vi "E709_Sample_Application_1.vi"() -> ()   [LabVIEW 2014, in "PiFOC.lvlib"]
doc: "This VI demonstrates how to initialize an E-709 system, how to move the axis and how to query for the position value of the axis. \n\nIn this example the E-709 is connected through COM port 1 with baudrate 115200. The VI runs E709_Configuration_Setup.vi with these specified settings, moves the axis relative to its current position and reads the position of the axis. The diagram shows how to combine the driver VIs for these tasks. \n\nWarning: Before running this VI, modify the \"Interface\" and \"RS232 settings\" (or \"USB settings\") to reflect your configuration. The predefined settings provided with the VI probably do not match your system."
uses:
  PiFOC.lvlib
panel:
  in  "stop":bool
  in  "error in":errorcluster
  out "Running":bool caption="Configuration_Setup.vi is running"
  out "error out":errorcluster
  out "Position":dbl[](array[numeric]) format="%.6f"
  out "Conn. axis":string[](array[string])
  out "Identification":string
  # "This VI demonstrates how to initialize an E-709 system, how to move an axis and how to query for the position value of this axis. \nThe VI runs E709_Configuration_Setup.vi with specified settings, moves the first axis relative to its current position and reads the\nposition of this axis. The diagram shows how to combine the driver VIs for these tasks. \n\nWarning: Before running this VI, modify the interface settings on the block diagram to reflect your configuration. The predefined \n                 settings provided with the VI probably do not match your system."
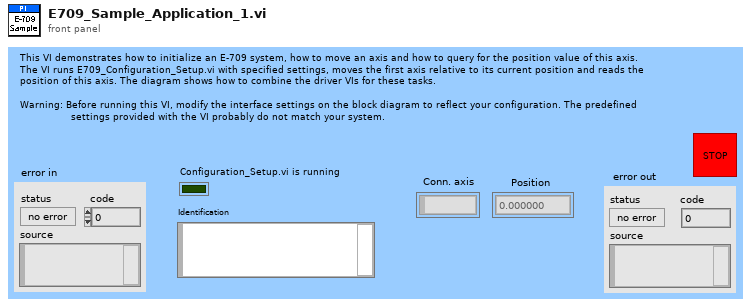
[diagram p1: front panel]
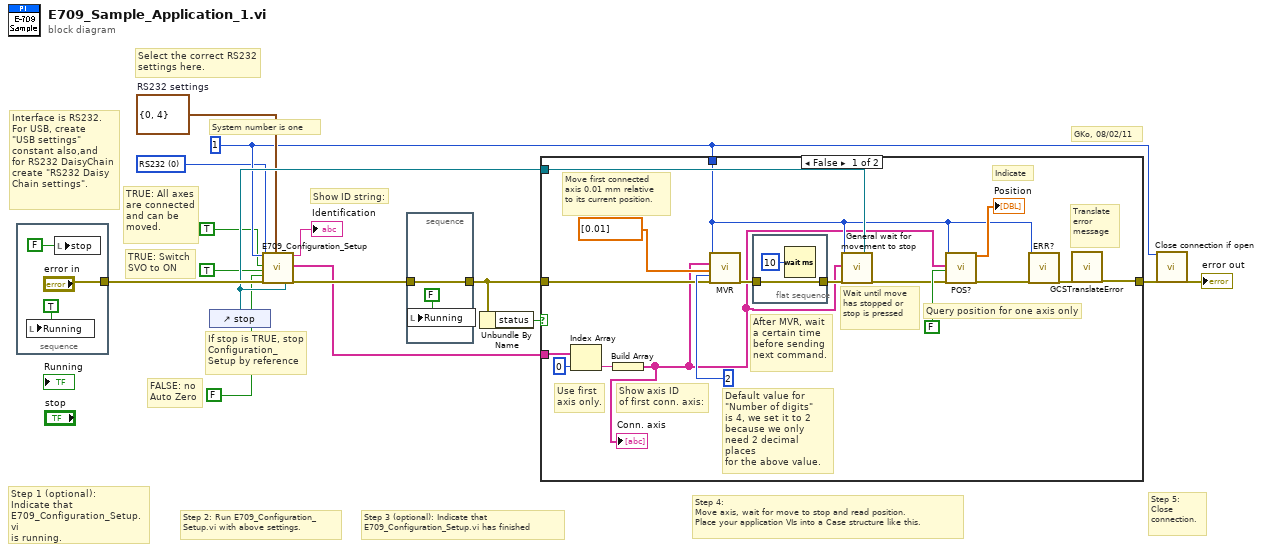
[diagram p0: block diagram]
diagram:
  w1 = u16 0 items=["RS232", "USB", "RS232 DaisyChain"] ("Interface")
  w8 = cluster{"Portnumber":i32, "Baudrate":u16} {"Portnumber"=0, "Baudrate"=4}  # RS232 settings
  w5 = 1 ("System no.")
  # "FALSE: no\nAuto Zero"
  # "Step 5: \nClose\nconnection."
  # "Interface is RS232.\nFor USB, create \n\"USB settings\"\nconstant also,and \nfor RS232 DaisyChain\ncreate \"RS232 Daisy\nChain settings\"."
  # "TRUE: All axes\nare connected\nand can be\nmoved."
  # "TRUE: Switch\nSVO to ON"
  # "If stop is TRUE, stop\nConfiguration_\nSetup by reference"
  # "Step 4: \nMove axis, wait for move to stop and read position.\nPlace your application VIs into a Case structure like this."
  # "Select the correct RS232\nsettings here."
  # "GKo, 08/02/11"
  # "Step 3 (optional): Indicate that \nE709_Configuration_Setup.vi has finished"
  # "Step 2: Run E709_Configuration_\nSetup.vi with above settings."
  # "Step 1 (optional): \nIndicate that \nE709_Configuration_Setup.vi\nis running."
  # "Show ID string:"
  # "System number is one"
  n1 = stacked-sequence {
    tunnel: ["error in"] -> w13
    frame #0 {
      n2 = local write "Running"(TRUE ("Running")) -> ()
      n3 = local write "stop"(FALSE ("stop")) -> ()
    }
  }
  n4 = control-ref of="stop"() -> (w10:refnum<vi>)
  n5 = call "E709_Configuration_Setup.vi"("System no."=w5, "Interface"=w1, "Connected?"=TRUE ("All axes?"), "Change servo status to ON?"=TRUE ("Use dialog to define\nconnected stages?"), "Perform autozero?"=FALSE, "error in"=w13, "RS232 settings"=w8, "Stop refnum"=w10) -> ("Identification"=→"Identification":string, "Conn. \nAxis"=w9:string[], "error out"=w14:errorcluster)  [unwired: 6 in, 3 out]
  n6 = stacked-sequence {
    tunnel: w14 -> [w20]
    tunnel: [w20] -> w12
    frame #0 {
      n7 = local write "Running"(FALSE ("Running")) -> ()
    }
  }
  n8 = Unbundle By Name(w12) -> ("status"=w11:bool)
  n9 = case shown="False" w11 {
    tunnel: [w32 w40] -> w7
    tunnel: w9 -> [w24 _]
    tunnel: w5 -> [w28 _]
    tunnel: w12 -> [w33 w40]
    tunnel: w10 -> [w31 _]
    frame False {
      # "Show axis ID\nof first conn. axis:"
      # "Use first\naxis only."
      # "After MVR, wait\na certain time\nbefore sending\nnext command."
      # "Translate\nerror \nmessage"
      # "Wait until move\nhas stopped or\nstop is pressed"
      # "Indicate"
      # "Default value for\n\"Number of digits\"\nis 4, we set it to 2\nbecause we only\nneed 2 decimal places\nfor the above value."
      # "Move first connected\naxis 0.01 mm relative\nto its current position."
      # "Query position for one axis only"
      n10 = Index Array(array=w24, index=0) -> (element=w22:string)
      n11 = Build Array(w22) -> (w21:string[])
      "Conn. axis" <- w21
      n12 = call "MVR.vi"("System no."=w28, "Axes to move"=w21, "Position values"=dbl[] [0.01], "No.of digits"=i16 2, "error in"=w33) -> ("error out"=w26:errorcluster)  [unwired: 14 out]
      n13 = flat-sequence {
        tunnel: w26 -> [w39]
        tunnel: [w39] -> w25
        frame #0 {
          n14 = Wait (ms)(milliseconds to wait=u32 10) -> ()  [unwired: 1 out]
        }
      }
      n15 = call "General wait for movement to stop.vi"("System no."=w28, "Axes to wait for"=w21, "error in"=w25, "Stop refnum"=w31) -> ("error out"=w27:errorcluster)  [unwired: 4 in, 11 out]
      n16 = call "POS?.vi"("System no."=w28, "Axes to query"=w21, "All axes?"=FALSE, "error in"=w27) -> ("Position"=→"Position":dbl[], "error out"=w30:errorcluster)  [unwired: 1 in, 13 out]
      n17 = call "ERR?.vi"("System no."=w28, "error in"=w30) -> ("error out"=w29:errorcluster)  [unwired: 17 out]
      n18 = call "GCSTranslateError.vi"("error in"=w29) -> ("error out"=w32:errorcluster)  [unwired: 18 out]
    }
    frame True {
      # "Error during initialization"
    }
  }
  n19 = call "Close connection if open.vi"("System no."=w5, "error in"=w7) -> ("error out"=→"error out":errorcluster)  [unwired: 1 in, 16 out]
